vi "Open VI.vi"(8 "error in (no error)":errorcluster, 11 "PrintToSingleFileHtml in":refnum<class "PrintToSingleFileHtml.lvclass">) -> (0 "error out":errorcluster, 2 "VI reference":refnum<vi>, 3 "PrintToSingleFileHtml out":refnum<class "PrintToSingleFileHtml.lvclass">)   [LabVIEW 2026, in "PrintToSingleFileHtml.lvclass"]
uses:
  PrintToSingleFileHtml.lvclass
  PrintToSingleFileHtml.lvclass/PrintToSingleFileHtml.ctl
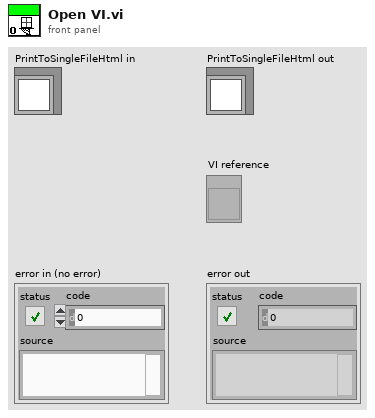
[diagram p1: front panel]
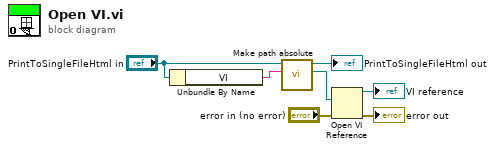
[diagram p0: block diagram]
diagram:
  n1 = Unbundle By Name("PrintToSingleFileHtml in") -> ("VI"=w6:string)
  n2 = call "Make path absolute.vi"("relative or absolute path"=w6, "PrintToSingleFileHtml in"="PrintToSingleFileHtml in") -> ("absolute path"=w2:path, "PrintToSingleFileHtml out"=→"PrintToSingleFileHtml out":refnum<class "PrintToSingleFileHtml.lvclass">)  [unwired: 8 in]
  n3 = Open VI Reference(vi path=w2, error in (no error)="error in (no error)") -> (vi reference=→"VI reference":refnum<vi>, error out=→"error out":errorcluster)  [unwired: 4 in]
